vi "Loop_SM.vi"() -> ()   [LabVIEW 2017, in "Climber.lvlib"]
uses:
  Climber.lvlib
  TypeDefs/Cluster_SRX Status No Encoder.ctl
  ENUM_State.ctl
  ENUM_Action.ctl
  Cluster_Cmd to SM Data.ctl
  ENUM_SM Cmd Select.ctl
  Globals/Global_STOP.vi
  Global_CMD to SM Data.vi
  Global_HW_Status.vi
  Global_SM_Data Out.vi
panel:
  out "Pitch":dbl
  out "HW_Climber_Status":T1
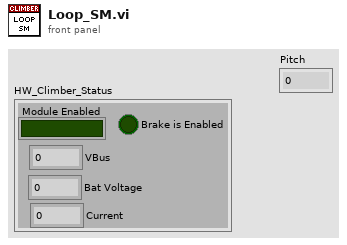
[diagram p1: front panel]
types:
  T1 = typedef "Cluster_SRX Status No Encoder.ctl" = cluster{"VBus ":dbl, "Module Enabled":bool, "Current":dbl, "Brake is Enabled":bool, "Bat Voltage":dbl}
  T2 = typedef "Climber.lvlib/Cluster_Cmd to SM Data.ctl" = cluster{"Climber Command Mode":T3}
  T3 = typedef "Climber.lvlib/ENUM_SM Cmd Select.ctl" = enum16{"Stop", "Auto Climb", "Manual", "No Command"}
  T4 = typedef "Climber.lvlib/ENUM_Action.ctl" = enum16{"No Action", "Auto Drive Climber", "Drive Climber", "Reset All", "Slow Climb", "Fast Climb"}
  T5 = typedef "Climber.lvlib/ENUM_State.ctl" = enum16{"Auto Rope Engage", "Auto Rope Climb", "Manual Speed Control", "No command", "Startup", "Idle", "Shutdown"}
  T6 = cluster{"Actions":T4[], "State":T5, "Current Time":timestamp, "Start Time":timestamp, "Loop Time (ms)":u32, "Climber Cmd":T2, "Climber Vbus OUT":dbl, "HW_Status":T1, "Gyro Angle":dbl}
  T7 = cluster{"Yaw":dbl, "Roll":dbl, "Pitch":dbl, "Heading":dbl, "Fused Heading":dbl}
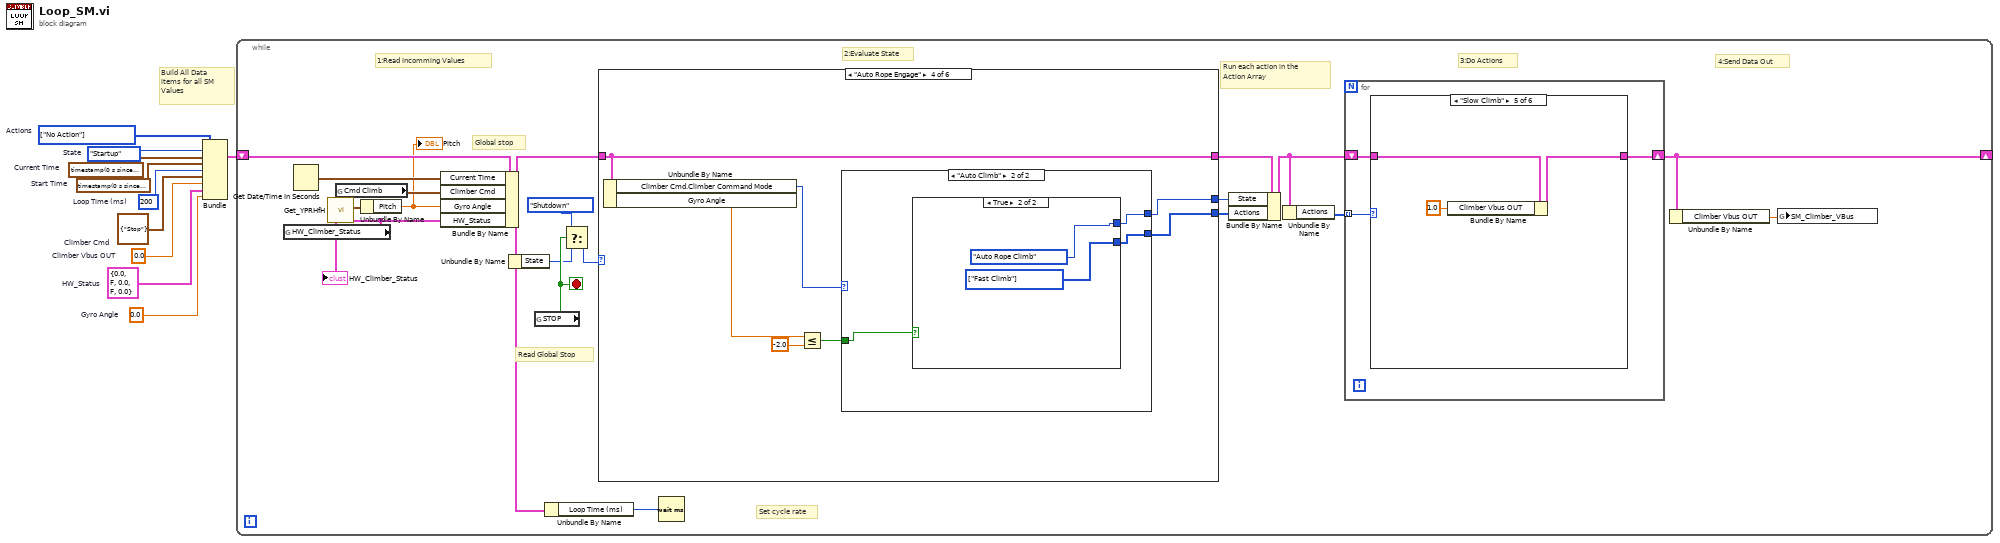
[diagram p0: block diagram]
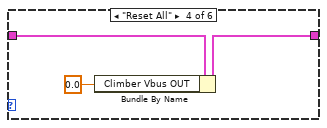
[diagram p5: hidden frame]
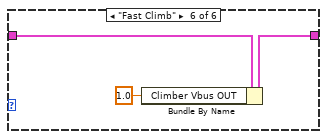
[diagram p6: hidden frame]
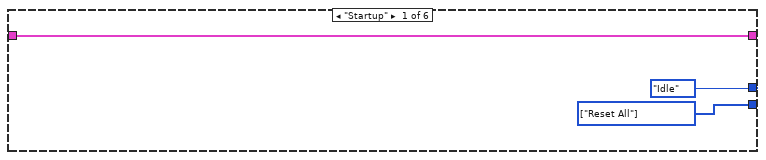
[diagram p7: hidden frame]
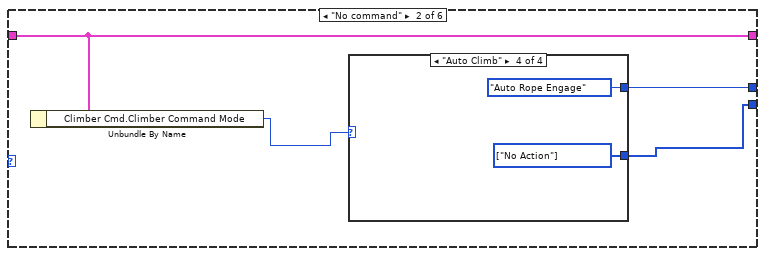
[diagram p8: hidden frame]
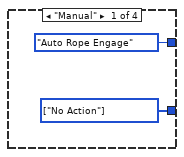
[diagram p9: hidden frame]
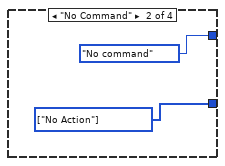
[diagram p10: hidden frame]
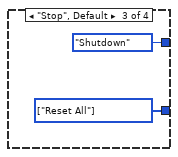
[diagram p11: hidden frame]
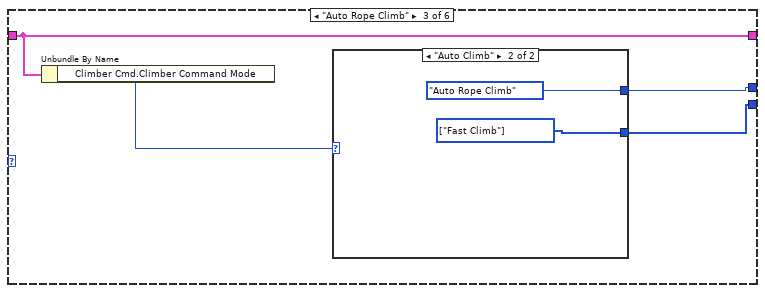
[diagram p12: hidden frame]
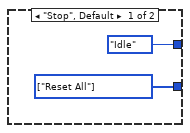
[diagram p13: hidden frame]
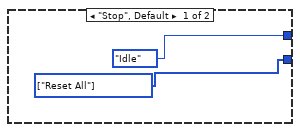
[diagram p14: hidden frame]
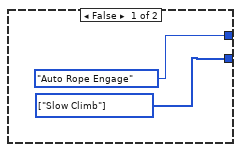
[diagram p15: hidden frame]
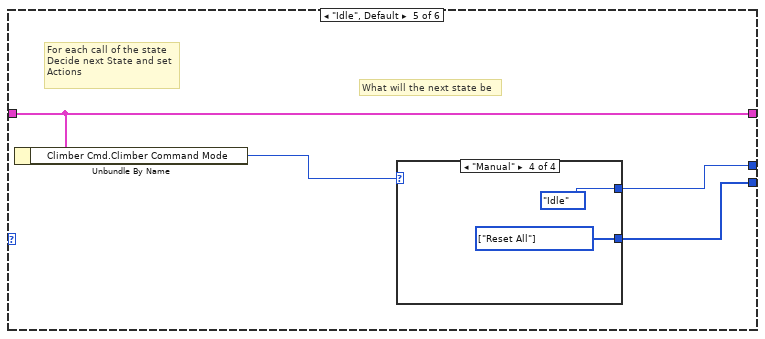
[diagram p16: hidden frame]
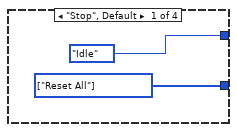
[diagram p17: hidden frame]
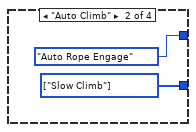
[diagram p18: hidden frame]
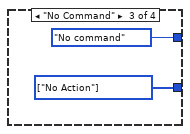
[diagram p19: hidden frame]
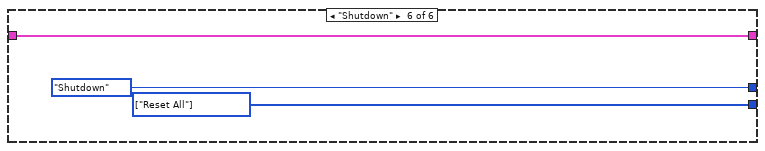
[diagram p20: hidden frame]
diagram:
  w1 = 0.0  # Gyro Angle
  w2 = T1 {"VBus "=0.0, "Module Enabled"=FALSE, "Current"=0.0, "Brake is Enabled"=FALSE, "Bat Voltage"=0.0}  # HW_Status
  w3 = 0.0  # Climber Vbus OUT
  w4 = T2 {"Climber Command Mode"=enum."Stop"}  # Climber Cmd
  w5 = u32 200  # Loop Time (ms)
  w6 = T4[] [enum."No Action"] items=["No Action", "Auto Drive Climber", "Drive Climber", "Reset All", "Slow Climb", "Fast Climb"]  # Actions
  w7 = timestamp(0 s since 1904-01-01)  # Start Time
  w8 = timestamp(0 s since 1904-01-01)  # Current Time
  w9 = ENUM_State."Startup"  # State
  # "Build All Data items for all SM Values"
  n1 = Bundle("Actions"=w6, "State"=w9, "Current Time"=w8, "Start Time"=w7, "Loop Time (ms)"=w5, "Climber Cmd"=w4, "Climber Vbus OUT"=w3, "HW_Status"=w2, "Gyro Angle"=w1) -> (w10:T6)  [unwired: 1 in]
  n2 = while {
    shift-right: [w18] -> _
    shift-left: w10 -> [w28]
    stop <- w22 stop-if-true
    # "Set cycle rate"
    # "Run each action in the Action Array"
    # "Read Global Stop"
    # "1:Read Incomming Values"
    # "2:Evaluate State"
    # "3:Do Actions"
    # "4:Send Data Out"
    # "Global stop"
    n3 = global read "Global_HW_Status.vi" "HW_Climber_Status"() -> (w13:T1)
    "HW_Climber_Status" <- w13
    n4 = Get Date/Time In Seconds() -> (seconds since 1Jan1904=w27:timestamp)
    n5 = call <vilib>:"Get_YPRHfH.vi"() -> ("YRPHfH"=w14:T7)  [unwired: 11 in]
    n6 = global read "Global_CMD to SM Data.vi" "Cmd Climb"() -> (w15:T2)
    n7 = Unbundle By Name(w14) -> ("Pitch"=w11:dbl)
    "Pitch" <- w11
    n8 = Bundle By Name(cluster=w28, "Current Time"=w27, "Climber Cmd"=w15, "Gyro Angle"=w11, "HW_Status"=w13) -> (w16:T6)
    n9 = Unbundle By Name(w16) -> ("State"=w20:T5)
    n10 = global read "Global_Stop.vi" "STOP"() -> (w22:bool)
    n11 = Unbundle By Name(w16) -> ("Loop Time (ms)"=w17:u32)
    n12 = Select(t=ENUM_State."Shutdown" ("State"), s=w22, f=w20) -> (s? t:f=w19:T5)
    n13 = case shown="\"Auto Rope Engage\"" w19 {
      tunnel: w16 -> [w47 w51 w63 w74 w86 w98]
      tunnel: [w47 w51 w63 w74 w86 w98] -> w25
      tunnel: [ENUM_State."Idle" ("State") w49 w61 w72 w87 ENUM_State."Shutdown" ("State")] -> w24
      tunnel: [w45 w48 w60 w71 w84 w96] -> w23
      frame "Startup" {
        w45 = T4[] [enum."Reset All"] items=["No Action", "Auto Drive Climber", "Drive Climber", "Reset All", "Slow Climb", "Fast Climb"] ("Actions")
      }
      frame "No command" {
        n14 = Unbundle By Name(w51) -> ("Climber Cmd.Climber Command Mode"=w50:T3)
        n15 = case shown="\"Auto Climb\"" w50 {
          tunnel: [ENUM_State."Auto Rope Engage" ("State") ENUM_State."No command" ("State") ENUM_State."Shutdown" ("State") ENUM_State."Auto Rope Engage" ("State")] -> w49
          tunnel: [w52 w54 w56 w58] -> w48
          frame "Manual" {
            w52 = T4[] [enum."No Action"] items=["No Action", "Auto Drive Climber", "Drive Climber", "Reset All", "Slow Climb", "Fast Climb"] ("Actions")
          }
          frame "No Command" {
            w54 = T4[] [enum."No Action"] items=["No Action", "Auto Drive Climber", "Drive Climber", "Reset All", "Slow Climb", "Fast Climb"] ("Actions")
          }
          frame "Stop", Default {
            w56 = T4[] [enum."Reset All"] items=["No Action", "Auto Drive Climber", "Drive Climber", "Reset All", "Slow Climb", "Fast Climb"] ("Actions")
          }
          frame "Auto Climb" {
            w58 = T4[] [enum."No Action"] items=["No Action", "Auto Drive Climber", "Drive Climber", "Reset All", "Slow Climb", "Fast Climb"] ("Actions")
          }
        }
      }
      frame "Auto Rope Climb" {
        n16 = Unbundle By Name(w63) -> ("Climber Cmd.Climber Command Mode"=w62:T3)
        n17 = case shown="\"Auto Climb\"" w62 {
          tunnel: [ENUM_State."Idle" ("State") ENUM_State."Auto Rope Climb" ("State")] -> w61
          tunnel: [w64 w66] -> w60
          frame "Stop", Default {
            w64 = T4[] [enum."Reset All"] items=["No Action", "Auto Drive Climber", "Drive Climber", "Reset All", "Slow Climb", "Fast Climb"] ("Actions")
          }
          frame "Auto Climb" {
            w66 = T4[] [enum."Fast Climb"] items=["No Action", "Auto Drive Climber", "Drive Climber", "Reset All", "Slow Climb", "Fast Climb"] ("Actions")
          }
        }
      }
      frame "Auto Rope Engage" {
        n18 = Unbundle By Name(w74) -> ("Climber Cmd.Climber Command Mode"=w73:T3, "Gyro Angle"=w68:dbl)
        n19 = Less Or Equal?(x=w68, y=-2.0) -> (x <= y?=w69:bool)
        n20 = case shown="\"Auto Climb\"" w73 {
          tunnel: [ENUM_State."Idle" ("State") w79] -> w72
          tunnel: [w75 w78] -> w71
          tunnel: w69 -> [_ w77]
          frame "Stop", Default {
            w75 = T4[] [enum."Reset All"] items=["No Action", "Auto Drive Climber", "Drive Climber", "Reset All", "Slow Climb", "Fast Climb"] ("Actions")
          }
          frame "Auto Climb" {
            n21 = case shown="True" w77 {
              tunnel: [ENUM_State."Auto Rope Engage" ("State") ENUM_State."Auto Rope Climb" ("State")] -> w79
              tunnel: [w80 w82] -> w78
              frame False {
                w80 = T4[] [enum."Slow Climb"] items=["No Action", "Auto Drive Climber", "Drive Climber", "Reset All", "Slow Climb", "Fast Climb"] ("Actions")
              }
              frame True {
                w82 = T4[] [enum."Fast Climb"] items=["No Action", "Auto Drive Climber", "Drive Climber", "Reset All", "Slow Climb", "Fast Climb"] ("Actions")
              }
            }
          }
        }
      }
      frame "Idle", Default {
        # "For each call of the state\nDecide next State and set\nActions"
        # "What will the next state be"
        n22 = Unbundle By Name(w86) -> ("Climber Cmd.Climber Command Mode"=w85:T3)
        n23 = case shown="\"Manual\"" w85 {
          tunnel: [ENUM_State."Idle" ("State") ENUM_State."Auto Rope Engage" ("State") ENUM_State."No command" ("State") ENUM_State."Idle" ("State")] -> w87
          tunnel: [w88 w90 w92 w94] -> w84
          frame "Stop", Default {
            w88 = T4[] [enum."Reset All"] items=["No Action", "Auto Drive Climber", "Drive Climber", "Reset All", "Slow Climb", "Fast Climb"] ("Actions")
          }
          frame "Auto Climb" {
            w90 = T4[] [enum."Slow Climb"] items=["No Action", "Auto Drive Climber", "Drive Climber", "Reset All", "Slow Climb", "Fast Climb"] ("Actions")
          }
          frame "No Command" {
            w92 = T4[] [enum."No Action"] items=["No Action", "Auto Drive Climber", "Drive Climber", "Reset All", "Slow Climb", "Fast Climb"] ("Actions")
          }
          frame "Manual" {
            w94 = T4[] [enum."Reset All"] items=["No Action", "Auto Drive Climber", "Drive Climber", "Reset All", "Slow Climb", "Fast Climb"] ("Actions")
          }
        }
      }
      frame "Shutdown" {
        w96 = T4[] [enum."Reset All"] items=["No Action", "Auto Drive Climber", "Drive Climber", "Reset All", "Slow Climb", "Fast Climb"] ("Actions")
      }
    }
    n24 = Wait (ms)(milliseconds to wait=w17) -> ()  [unwired: 1 out]
    n25 = Bundle By Name(cluster=w25, "State"=w24, "Actions"=w23) -> (w26:T6)
    n26 = Unbundle By Name(w26) -> ("Actions"=w29:T4[])
    n27 = for {
      tunnel: w29 -> [w32] mode=indexing
      shift-right: [w31] -> w18
      shift-left: w26 -> [w30]
      n28 = case shown="\"Slow Climb\"" w32 {
        tunnel: w30 -> [w33 w34 w35 w38 w41 w44]
        tunnel: [w33 w34 w35 w37 w40 w43] -> w31
        frame "No Action" {
        }
        frame "Drive Climber" {
          # "Reset timer by taking the current time\nand making it the start time\n\nLater when the current time is \nsubtracted from the start time\nyou will get the elapsed time in \nseconds"
        }
        frame "Auto Drive Climber" {
        }
        frame "Reset All" {
          n29 = Bundle By Name(cluster=w38, "Climber Vbus OUT"=0.0 ("Climber Speed")) -> (w37:T6)
        }
        frame "Slow Climb" {
          n30 = Bundle By Name(cluster=w41, "Climber Vbus OUT"=1.0) -> (w40:T6)
        }
        frame "Fast Climb" {
          n31 = Bundle By Name(cluster=w44, "Climber Vbus OUT"=1.0) -> (w43:T6)
        }
      }
    }
    n32 = Unbundle By Name(w18) -> ("Climber Vbus OUT"=w12:dbl)
    n33 = global write "Global_SM_Data Out.vi" "SM_Climber_VBus"(w12) -> ()
  }
